vi "Write Set DER SetPointF Msg.vi"(10 "Set DER SetPointF Msg":refnum<class "Set DER SetPointF Msg.lvclass">, 11 "SCADA Sub Abstract in":refnum<class "Device Communication and Control Abstract.lvclass">) -> (3 "SCADA Sub Abstract out":refnum<class "Device Communication and Control Abstract.lvclass">)   [LabVIEW 2018, in "Device Communication and Control Abstract Actor.lvlib" / "Device Communication and Control Abstract.lvclass"]
uses:
  Device Communication and Control Abstract.lvclass
  Device Communication and Control Abstract Messages/Set DER SetPointF Msg/Set DER SetPointF Msg.lvclass
  Device Communication and Control Abstract.lvclass/Device Communication and Control Abstract.ctl
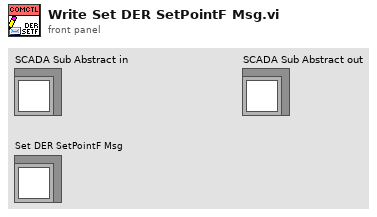
[diagram p1: front panel]
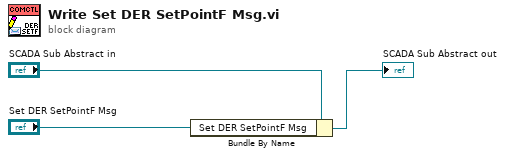
[diagram p0: block diagram]
diagram:
  n1 = Bundle By Name(cluster="SCADA Sub Abstract in", "Set DER SetPointF Msg"="Set DER SetPointF Msg") -> (→"SCADA Sub Abstract out":refnum<class "Device Communication and Control Abstract.lvclass">)
